vi "Construct_Optimal_Subtrack_101_2_Subtracks-1.vi"(0 "[IN] Still connected\ntracks in group":T2, 1 "[IN] Indexes for Jumps":i32[](array[numeric]), 5 "[IN] Clusters for Re\nconstructed Tracks":T1, 7 "[IN] Index of recon\nstructed tracks":i32, 11 "error IN":errorcluster, 12 "[IN] # column of op\ntimal elongation":i32, 13 "[IN] Indicies of Po\nints Inside Trks":i32[](array[numeric]), 14 "[IN] Indicies of all \nAffected Tracks \n(initial point = 0)":i32[](array[numeric])) -> (6 "[OUT] Clusters for Re\nconstructed Tracks":T1, 15 "error OUT":errorcluster)   [LabVIEW 2017]
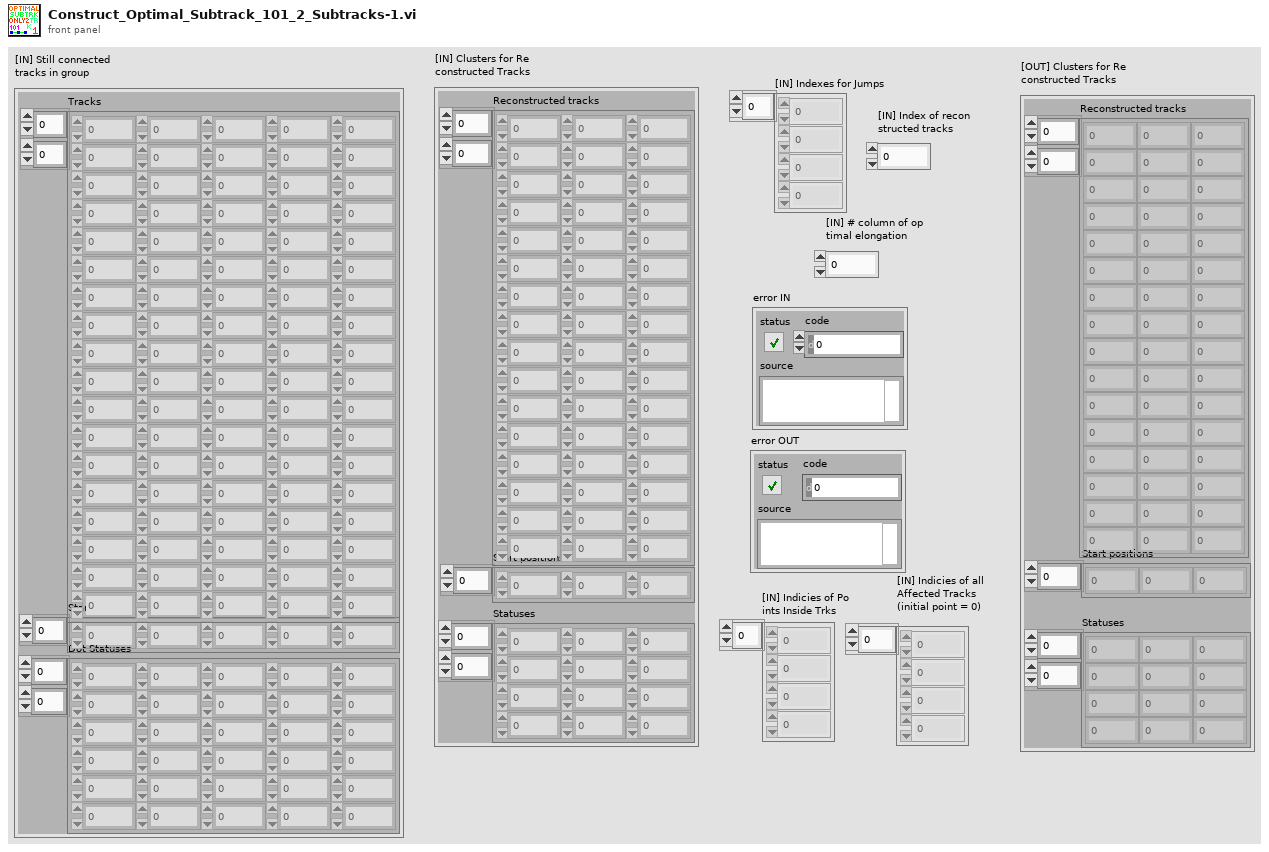
[diagram p1: front panel]
types:
  T1 = cluster{"Reconstructed tracks":dbl[][], "Start positions":i32[], "Statuses":i16[][]}
  T2 = cluster{"Tracks":dbl[][], "Start Pos":i32[], "Dot Statuses":i16[][]}
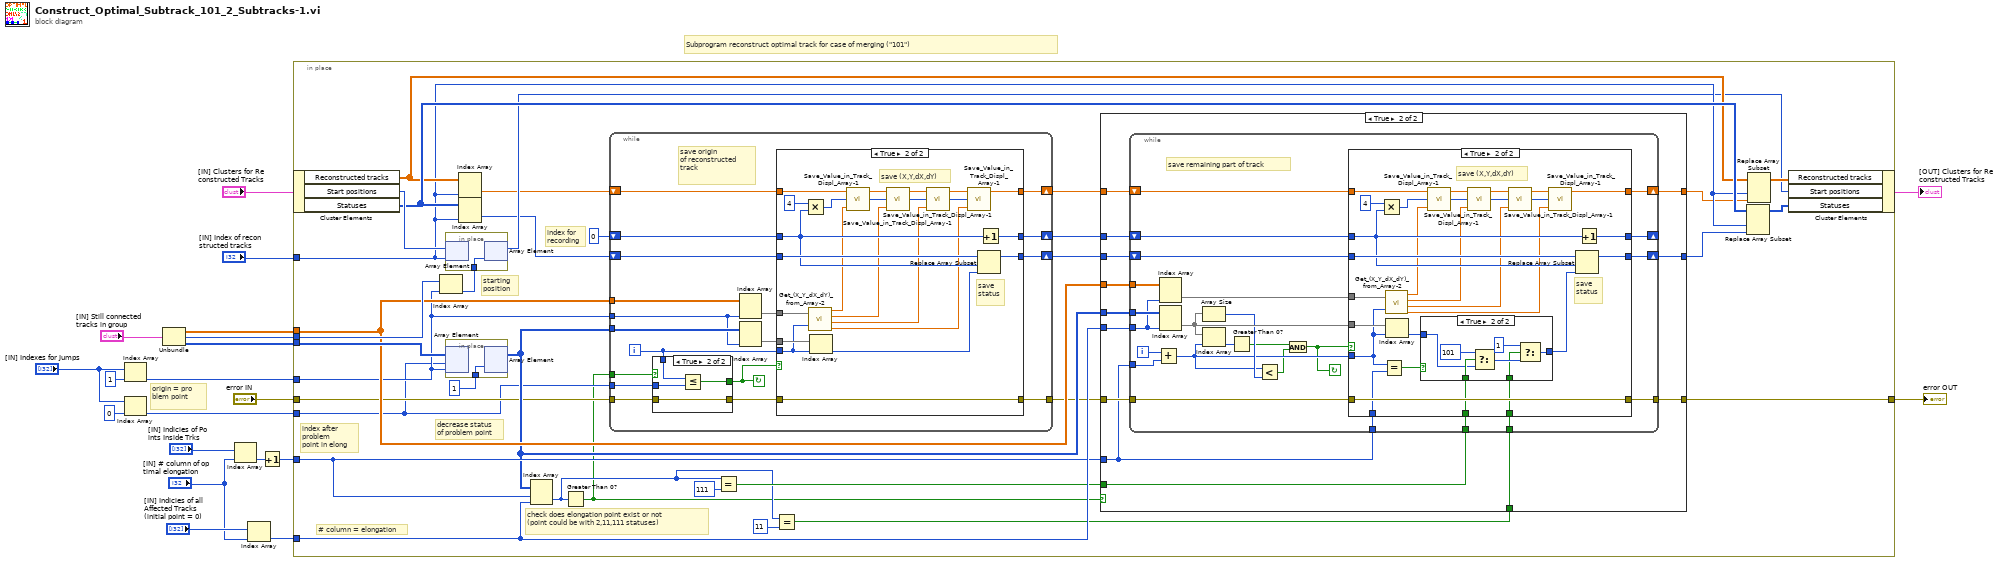
[diagram p0: block diagram]
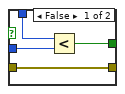
[diagram p2: hidden frame]
diagram:
  # "origin = pro\nblem point"
  # "Subprogram reconstruct optimal track for case of merging (\"101\")"
  n1 = Index Array(array="[IN] Indexes for Jumps", index=1) -> (element=w14:i32)
  n2 = Index Array(array="[IN] Indexes for Jumps", index=0) -> (element=w10:i32)
  n3 = Unbundle("[IN] Still connected\ntracks in group") -> ("Tracks"=w11:dbl[][], "Start Pos"=w12:i32[], "Dot Statuses"=w13:i16[][])
  n4 = Index Array(array="[IN] Indicies of Po\nints Inside Trks", index="[IN] # column of op\ntimal elongation") -> (element=w3:i32)
  n5 = Index Array(array="[IN] Indicies of all \nAffected Tracks \n(initial point = 0)", index="[IN] # column of op\ntimal elongation") -> (element=w5:i32)
  n6 = Increment(x=w3) -> (x+1=w2:i32)
  n7 = in-place {
    in-place-border: "[IN] Index of recon\nstructed tracks" -> [w50]
    in-place-border: w14 -> [w29]
    in-place-border: w13 -> [w38]
    in-place-border: w12 -> [w54]
    in-place-border: w11 -> [w30]
    in-place-border: w10 -> [w26]
    in-place-border: "error IN" -> [w27]
    in-place-border: w5 -> [w42]
    in-place-border: [w46] -> w7
    in-place-border: w2 -> [w41]
    # "decrease status\nof problem point"
    # "check does elongation point exist or not  \n(point could be with 2,11,111 statuses)"
    # "# column = elongation"
    # "index after\nproblem \npoint in elong"
    # "index for\nrecording"
    # "starting\nposition"
    n8 = in-place-cluster #1("[IN] Clusters for Re\nconstructed Tracks") -> ("Reconstructed tracks"=w51:dbl[][], "Start positions"=w53:i32[], "Statuses"=w52:i16[][])
    n9 = Index Array(array=w54, index=w29) -> (element=w45:i32)
    n10 = in-place {
      in-place-border: w45 -> [w189]
      n11 = in-place-array #2(w53, w50) -> ()  [unwired: 1 out]
      n12 = in-place-array #2(w189) -> (w48:i32[])  [unwired: 1 out]
    }
    n13 = in-place {
      in-place-border: i16 1 ("element") -> [w108]
      n14 = in-place-array #3(w38, w26, w29) -> ()  [unwired: 1 out]
      n15 = in-place-array #3(w108) -> (w28:i16[][])  [unwired: 2 out]
    }
    n16 = Index Array(array=w51, index (col)=w50) -> (element=w32:dbl[])  [unwired: 1 in]
    n17 = Index Array(array=w52, index (col)=w50) -> (element=w31:i16[])  [unwired: 1 in]
    n18 = Index Array(array=w28, index (row)=w41, index (col)=w42) -> (element=w35:i16)
    n19 = Greater Than 0?(x=w35) -> (x > 0?=w21:bool)
    n20 = while {
      tunnel: w26 -> [w58]
      tunnel: w30 -> [w72]
      tunnel: w28 -> [w71]
      tunnel: w29 -> [w70]
      shift-right: [w64] -> w25
      shift-left: w32 -> [w69]
      shift-right: [w62] -> w23
      shift-left: w31 -> [w66]
      shift-right: [w63] -> w24
      shift-left: 0 -> [w65]
      tunnel: w27 -> [w56]
      tunnel: [w61] -> w22
      tunnel: w21 -> [w60]
      i -> [w59]
      stop <- w57 continue-if-true
      # "save origin \nof reconstructed \ntrack"
      n21 = case shown="True" w60 {
        tunnel: w59 -> [w76 w80]
        tunnel: w58 -> [w75 w79]
        tunnel: [w74 w78] -> w57
        tunnel: w56 -> [w73 w77]
        tunnel: [w73 w77] -> w55
        frame False {
          n22 = Less?(x=w76, y=w75) -> (x < y?=w74:bool)
        }
        frame True {
          n23 = Less Or Equal?(x=w80, y=w79) -> (x <= y?=w78:bool)
        }
      }
      n24 = Index Array(array=w72, index (col)=w70) -> (element=w68:dbl[])  [unwired: 1 in]
      n25 = Index Array(array=w71, index (col)=w70) -> (element=w67:i16[])  [unwired: 1 in]
      n26 = case shown="True" w57 {
        tunnel: w69 -> [w84 w97]
        tunnel: w68 -> [_ w107]
        tunnel: w67 -> [_ w106]
        tunnel: w59 -> [_ w102]
        tunnel: w66 -> [w82 w104]
        tunnel: [w82 w101] -> w62
        tunnel: [w84 w86] -> w64
        tunnel: w65 -> [w83 w100]
        tunnel: [w83 w99] -> w63
        tunnel: w55 -> [w81 w98]
        tunnel: [w81 w98] -> w61
        frame False {
        }
        frame True {
          # "save (X,Y,dX,dY)"
          # "save\nstatus"
          n27 = Multiply(x=4, y=w100) -> (x*y=w95:i32)
          n28 = call "Get_(X_Y_dX_dY)_from_Array-2.vi"("(X,Y,dX,dY)"=w107, "Index of Displacement"=w102) -> ("X"=w96:dbl, "Y"=w92:dbl, "dX"=w90:dbl, "dY"=w87:dbl)
          n29 = Index Array(array=w106, index=w102) -> (element=w103:i16)
          n30 = call "Save_Value_in_Track_Displ_Array-1.vi"("[IN] Value"=w96, "[IN] Index"=w95, "[IN] Empty tracks\nfor points saving"=w97) -> ("[OUT] Index ++"=w93:i32, "[OUT Track with saved value"=w94:dbl[])  [unwired: 1 in]
          n31 = call "Save_Value_in_Track_Displ_Array-1.vi"("[IN] Value"=w92, "[IN] Index"=w93, "[IN] Empty tracks\nfor points saving"=w94) -> ("[OUT] Index ++"=w89:i32, "[OUT Track with saved value"=w91:dbl[])  [unwired: 1 in]
          n32 = call "Save_Value_in_Track_Displ_Array-1.vi"("[IN] Value"=w90, "[IN] Index"=w89, "[IN] Empty tracks\nfor points saving"=w91) -> ("[OUT] Index ++"=w85:i32, "[OUT Track with saved value"=w88:dbl[])  [unwired: 1 in]
          n33 = call "Save_Value_in_Track_Displ_Array-1.vi"("[IN] Value"=w87, "[IN] Index"=w85, "[IN] Empty tracks\nfor points saving"=w88) -> ("[OUT Track with saved value"=w86:dbl[])  [unwired: 1 in, 1 out]
          n34 = Replace Array Subset(array=w104, new element=w103, index=w100) -> (w101:i16[])
          n35 = Increment(x=w100) -> (x+1=w99:i32)
        }
      }
    }
    n36 = Equal?(x=w35, y=i16 111) -> (x = y?=w39:bool)
    n37 = Equal?(x=w35, y=i16 11) -> (x = y?=w34:bool)
    n38 = case shown="True" w21 {
      tunnel: w30 -> [_ w124]
      tunnel: [w109 w123] -> w46
      tunnel: w25 -> [w111 w122]
      tunnel: w24 -> [_ w121]
      tunnel: w23 -> [w110 w120]
      tunnel: w22 -> [w109 w119]
      tunnel: [w111 w118] -> w44
      tunnel: [w110 w117] -> w43
      tunnel: w28 -> [_ w116]
      tunnel: w42 -> [_ w115]
      tunnel: w41 -> [_ w113]
      tunnel: w39 -> [_ w114]
      tunnel: w34 -> [_ w112]
      frame False {
      }
      frame True {
        n39 = while {
          tunnel: w124 -> [w148]
          tunnel: w116 -> [w147]
          tunnel: w115 -> [w146]
          shift-right: [w141] -> w118
          shift-left: w122 -> [w145]
          shift-right: [w139] -> w117
          shift-left: w120 -> [w143]
          shift-right: [w140] -> _
          shift-left: w121 -> [w142]
          tunnel: w113 -> [w137]
          tunnel: w119 -> [w129]
          tunnel: [w128] -> w123
          tunnel: w113 -> [w127]
          tunnel: w114 -> [w126]
          tunnel: w112 -> [w125]
          i -> [w138]
          stop <- w130 continue-if-true
          # "save remaining part of track"
          n40 = Add(x=w138, y=w137) -> (x+y=w133:i32)
          n41 = Index Array(array=w148, index (col)=w146) -> (element=w144:dbl[])  [unwired: 1 in]
          n42 = Index Array(array=w147, index (col)=w146) -> (element=w136:i16[])  [unwired: 1 in]
          n43 = Array Size(array=w136) -> (size(s)=w134:i32)
          n44 = Index Array(array=w136, index=w133) -> (element=w135:i16)
          n45 = Greater Than 0?(x=w135) -> (x > 0?=w132:bool)
          n46 = Less?(x=w133, y=w134) -> (x < y?=w131:bool)
          n47 = And(x=w132, y=w131) -> (x .and. y?=w130:bool)
          n48 = case shown="True" w130 {
            tunnel: w145 -> [w152 w166]
            tunnel: w144 -> [_ w180]
            tunnel: w136 -> [_ w179]
            tunnel: w133 -> [_ w172]
            tunnel: w143 -> [w150 w177]
            tunnel: [w150 w176] -> w139
            tunnel: [w152 w154] -> w141
            tunnel: w142 -> [w151 w175]
            tunnel: [w151 w174] -> w140
            tunnel: w129 -> [w149 w173]
            tunnel: [w149 w173] -> w128
            tunnel: w127 -> [_ w171]
            tunnel: w126 -> [_ w167]
            tunnel: w125 -> [_ w153]
            frame False {
            }
            frame True {
              # "save (X,Y,dX,dY)"
              # "save\nstatus"
              n49 = Multiply(x=4, y=w175) -> (x*y=w165:i32)
              n50 = Equal?(x=w172, y=w171) -> (x = y?=w170:bool)
              n51 = call "Get_(X_Y_dX_dY)_from_Array-2.vi"("(X,Y,dX,dY)"=w180, "Index of Displacement"=w172) -> ("X"=w164:dbl, "Y"=w161:dbl, "dX"=w159:dbl, "dY"=w155:dbl)
              n52 = Index Array(array=w179, index=w172) -> (element=w169:i16)
              n53 = case shown="True" w170 {
                tunnel: w169 -> [w181 w186]
                tunnel: [w181 w184] -> w168
                tunnel: w167 -> [_ w188]
                tunnel: w153 -> [_ w182]
                frame False {
                }
                frame True {
                  n54 = Select(t=i16 101 ("element"), s=w188, f=w186) -> (s? t:f=w183:i16)
                  n55 = Select(t=i16 1 ("element"), s=w182, f=w183) -> (s? t:f=w184:i16)
                }
              }
              n56 = call "Save_Value_in_Track_Displ_Array-1.vi"("[IN] Value"=w164, "[IN] Index"=w165, "[IN] Empty tracks\nfor points saving"=w166) -> ("[OUT] Index ++"=w162:i32, "[OUT Track with saved value"=w163:dbl[])  [unwired: 1 in]
              n57 = call "Save_Value_in_Track_Displ_Array-1.vi"("[IN] Value"=w161, "[IN] Index"=w162, "[IN] Empty tracks\nfor points saving"=w163) -> ("[OUT] Index ++"=w158:i32, "[OUT Track with saved value"=w160:dbl[])  [unwired: 1 in]
              n58 = call "Save_Value_in_Track_Displ_Array-1.vi"("[IN] Value"=w159, "[IN] Index"=w158, "[IN] Empty tracks\nfor points saving"=w160) -> ("[OUT] Index ++"=w156:i32, "[OUT Track with saved value"=w157:dbl[])  [unwired: 1 in]
              n59 = call "Save_Value_in_Track_Displ_Array-1.vi"("[IN] Value"=w155, "[IN] Index"=w156, "[IN] Empty tracks\nfor points saving"=w157) -> ("[OUT Track with saved value"=w154:dbl[])  [unwired: 1 in, 1 out]
              n60 = Replace Array Subset(array=w177, new element=w168, index=w175) -> (w176:i16[])
              n61 = Increment(x=w175) -> (x+1=w174:i32)
            }
          }
        }
      }
    }
    n62 = Replace Array Subset(array=w52, new element=w43, index (col)=w50) -> (w47:i16[][])  [unwired: 1 in]
    n63 = Replace Array Subset(array=w51, new element=w44, index (col)=w50) -> (w49:dbl[][])  [unwired: 1 in]
    n64 = in-place-cluster #1("Reconstructed tracks"=w49, "Start positions"=w48, "Statuses"=w47) -> (→"[OUT] Clusters for Re\nconstructed Tracks":T1)
  }
  "error OUT" <- w7
